vi "IAmGLF-NotARefnum.vi"(11 "IAmGLF in":refnum<class "IAmGLF.lvclass">) -> (2 "Not A Valid Refnum?":bool=TRUE, 3 "IAmGLF out":refnum<class "IAmGLF.lvclass">)   [LabVIEW 2020, in "GLF.lvlib" / "IAmGLF.lvclass"]
doc: "<B>Summary</B>\nReturns <B>True</B> if the class is invalid."
uses:
  IAmGLF.lvclass
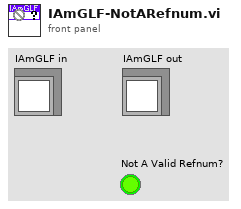
[diagram p1: front panel]
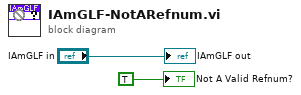
[diagram p0: block diagram]
diagram:
  "IAmGLF out" <- "IAmGLF in"
  "Not A Valid Refnum?" <- TRUE ("Not A Valid Refnum?")
